vi "Control_BSA_setup.vi"(0 "setup":T1, 7 "BSA number":string) -> ()   [LabVIEW 2011]
uses:
  Controls/Setup.ctl
  Globals/LDA_meas_global_2.vi
  Globals/LDA_meas_global_1.vi
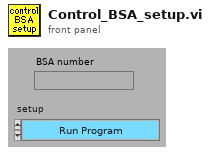
[diagram p1: front panel]
types:
  T1 = typedef "Setup.ctl" = enum16{"Run Program", "Show Setup", "Save Current Setup", "Setup Front Panel"}
  T2 = enum16{"Velocity", "Transit time", "Arrival time"}
  T3 = typedef "BSA_info_Cluster.ctl" = cluster{"GPIB Address":string, "No of Check Bytes":i32, "Extra Info":string, "COLOUR":u32, "Wavelength (nm)":dbl}
  T4 = cluster{"Output data format":enum16{"Velocity, transit time, arrival time", "Velocity, arrival time", "Velocity, transit time", "Velocity"}, "Non-validated signals":enum16{"Accept", "Reject"}}
  T5 = cluster{"High voltage":i16, "Signal gain (dB)":i16}
  T6 = enum16{"6.4", "3.2", "1.6", "0.8", "0.4", "0.2", "0.1", "0.05"}
  T7 = cluster{"Centre Velocity":u16, "Velocity span":u16, "Units":enum16{"Hz", "m/s"}, "Frequency shift":enum16{"Disabled", "Enabled"}}
  T8 = cluster{"Arrival time clock":enum16{"External", "Internal"}, "Clock source":enum16{"Slave", "Master", "Private"}, "Coincidence":enum16{"Slave", "Master", "Private"}}
  T9 = cluster{"Dead time (s)":dbl, "Duty cycle (%)":dbl, "Data collection mode":enum16{"Burst", "Contiuous", "Dead time", "External"}}
  T10 = cluster{"Burst criterion":enum16{"Envelope", "Pedestal", "Env and ped"}, "Oversize reject level":enum16{"1 (disabled)", "2", "3", "4", "5", "6", "7", "8", "9"}, "Pedestal attenuation":enum16{"0", "6", "12", "18"}, "Record length":enum16{"8", "16", "32", "64"}, "Quality factor":i16}
  T11 = cluster{"Centre frequency":u16, "Bandwidth":u16, "Units":enum16{"Hz", "m/s"}, "Frequency shift":enum16{"Disabled", "Enabled"}}
  T12 = enum16{"Velocity, transit time, arrival time", "Velocity, arrival time", "Velocity, transit time", "Velocity"}
  T13 = enum16{"Velocity", "Transit time", "Arrival time"}[]
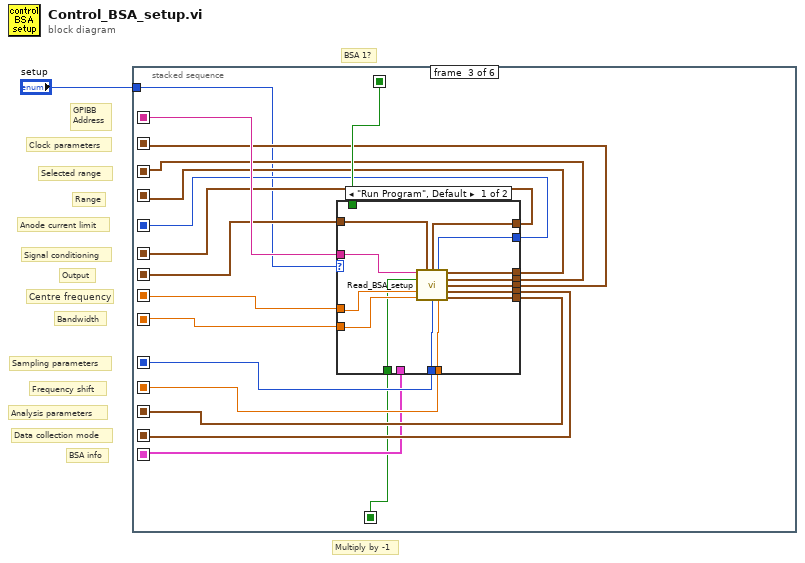
[diagram p0: block diagram]
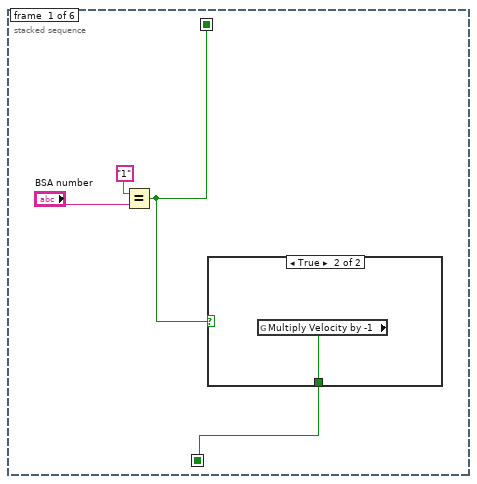
[diagram p2: hidden frame]
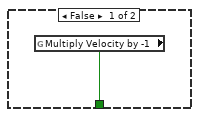
[diagram p3: hidden frame]
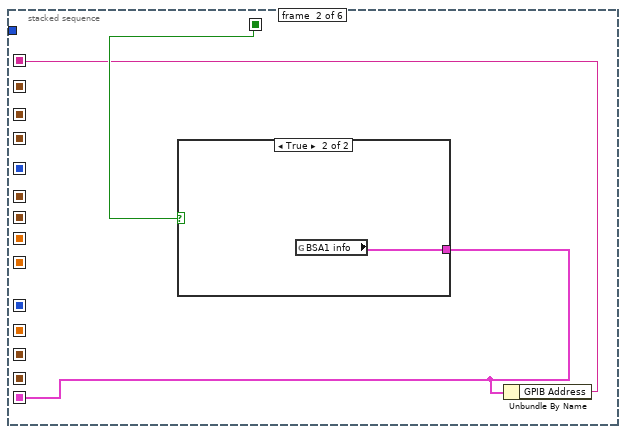
[diagram p4: hidden frame]
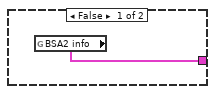
[diagram p5: hidden frame]
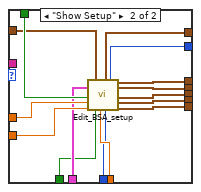
[diagram p6: hidden frame]
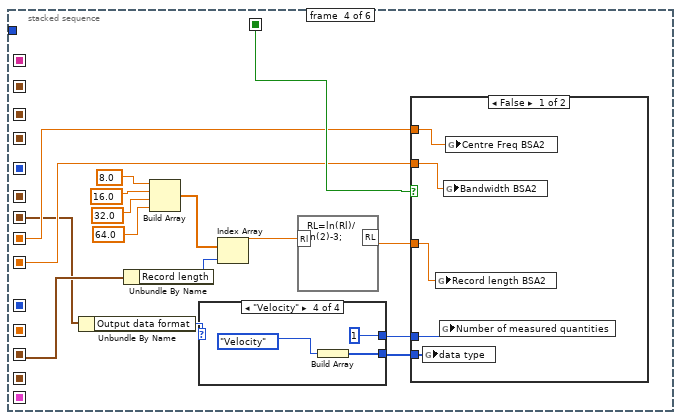
[diagram p7: hidden frame]
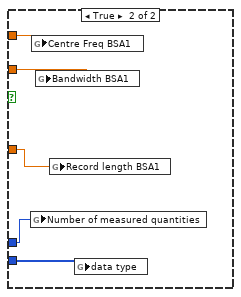
[diagram p8: hidden frame]
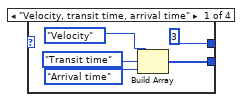
[diagram p9: hidden frame]
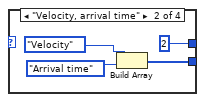
[diagram p10: hidden frame]
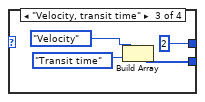
[diagram p11: hidden frame]
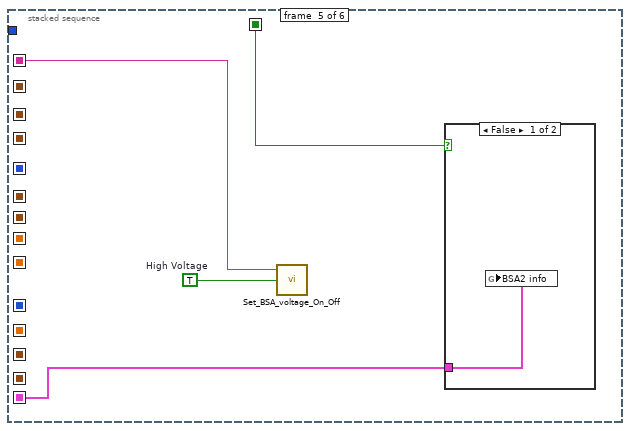
[diagram p12: hidden frame]
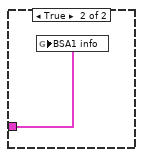
[diagram p13: hidden frame]
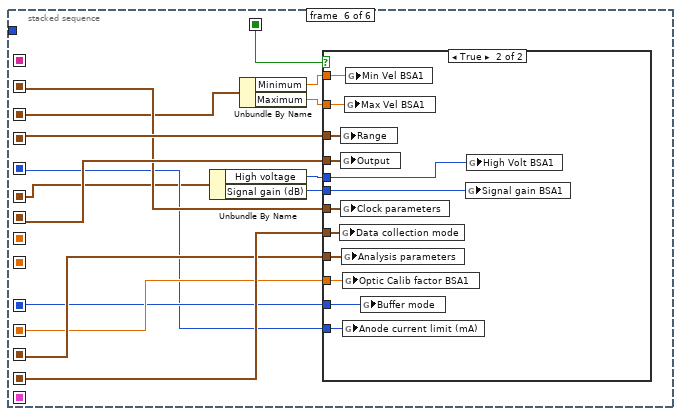
[diagram p14: hidden frame]
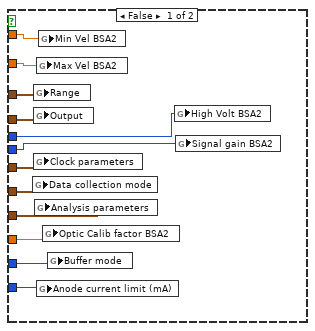
[diagram p15: hidden frame]
diagram:
  # "Multiply by -1"
  # "Bandwidth"
  # "Centre frequency"
  # "Anode current limit"
  # "Selected range"
  # "Range"
  # "Signal conditioning"
  # "Analysis parameters"
  # "Data collection mode"
  # "Frequency shift"
  # "Output"
  # "Clock parameters"
  # "Sampling parameters"
  # "BSA 1?"
  # "BSA info"
  # "GPIBB\nAddress"
  n1 = stacked-sequence {
    seq-local: [_ _ w27 _ _ _] -> [_ _ _ _ _ w117]
    seq-local: [_ w8 _ _ _ _] -> [_ _ w29 _ w101 _]
    seq-local: [_ w9 _ _ _ _] -> [_ _ w15 _ w104 _]
    seq-local: [w3 _ _ _ _ _] -> [_ w10 w28 w69 w103 w121]
    seq-local: [_ _ w20 _ _ _] -> [_ _ _ _ _ w109]
    seq-local: [_ _ w21 _ _ _] -> [_ _ _ _ _ w120]
    seq-local: [_ _ w22 _ _ _] -> [_ _ _ _ _ w113]
    seq-local: [_ _ w23 _ _ _] -> [_ _ _ _ _ w112]
    seq-local: [_ _ w24 _ _ _] -> [_ _ _ _ _ w114]
    seq-local: [_ _ w25 _ _ _] -> [_ _ _ _ _ w115]
    seq-local: [_ _ w26 _ _ _] -> [_ _ _ w66 _ w116]
    seq-local: [_ _ w19 _ _ _] -> [_ _ _ _ _ w118]
    seq-local: [_ _ w18 _ _ _] -> [_ _ _ w59 _ w119]
    seq-local: [_ _ w17 _ _ _] -> [_ _ _ w68 _ _]
    seq-local: [_ _ w16 _ _ _] -> [_ _ _ w67 _ _]
    seq-local: [w2 _ _ _ _ _] -> [_ _ w13 _ _ _]
    tunnel: "setup" -> [_ _ w14 _ _ _]
    frame #0 {
      n2 = Equal?(x="1", y="BSA number") -> (x = y?=w3:bool)
      n3 = case shown="True" w3 {
        tunnel: [w6 w7] -> w2
        frame False {
          n4 = global read "LDA_meas_global_2.vi" "Multiply Velocity by -1"() -> (w6:bool)
        }
        frame True {
          n5 = global read "LDA_meas_global_1.vi" "Multiply Velocity by -1"() -> (w7:bool)
        }
      }
    }
    frame #1 {
      n6 = case shown="True" w10 {
        tunnel: [w11 w12] -> w9
        frame False {
          n7 = global read "LDA_meas_global_2.vi" "BSA2 info"() -> (w11:T3)
        }
        frame True {
          n8 = global read "LDA_meas_global_1.vi" "BSA1 info"() -> (w12:T3)
        }
      }
      n9 = Unbundle By Name(w9) -> ("GPIB Address"=w8:string)
    }
    frame #2 {
      n10 = case shown="\"Run Program\", Default" w14 {
        tunnel: w29 -> [w43 _]
        tunnel: w28 -> [_ w58]
        tunnel: [w42 w57] -> w21
        tunnel: [w41 w56] -> w20
        tunnel: [w40 w55] -> w19
        tunnel: [w39 w54] -> w27
        tunnel: [w38 w53] -> w26
        tunnel: [w37 w52] -> w25
        tunnel: [w36 w51] -> w24
        tunnel: [w35 w50] -> w23
        tunnel: [w34 w49] -> w22
        tunnel: [w33 w48] -> w18
        tunnel: [w32 w47] -> w17
        tunnel: [w31 w46] -> w16
        tunnel: w15 -> [_ w45]
        tunnel: w13 -> [w30 w44]
        frame "Run Program", Default {
          n11 = call "Read_BSA_setup.vi"("GPIB Address"=w43, "Multiply Velocity by -1"=w30) -> ("Output"=w33:T4, "Signal conditioning"=w35:T5, "Anode current limit (mA)"=w34:T6, "Range"=w42:T7, "Selected range"=w41:cluster{"Minimum":dbl, "Maximum":dbl}, "Clock parameters"=w40:T8, "Centre frequency"=w32:dbl, "Data collection mode"=w39:T9, "Bandwidth"=w31:dbl, "Buffer mode"=w36:enum16{"One shot", "Ring", "FIFO"}, "Calibration factor"=w37:dbl, "Analysis parameters"=w38:T10)  [unwired: 1 in, 1 out]
        }
        frame "Show Setup" {
          n12 = call "Edit_BSA_setup.vi"("BSA info"=w45, "BSA 1?"=w58, "Multiply Velocity by -1"=w44) -> ("Centre frequency"=w47:dbl, "Bandwidth"=w46:dbl, "Output"=w48:T4, "Calibration factor"=w52:dbl, "Signal conditioning (out)"=w50:T5, "Buffer mode out"=w51:enum16{"One shot", "Ring", "FIFO"}, "Anode current limit (mA)"=w49:T6, "Range (out)"=w57:T11, "Selected range"=w56:cluster{"Minimum":dbl, "Maximum":dbl}, "Clock parameters (out)"=w55:T8, "Data collection mode (out)"=w54:T9, "Analysis parameters (out)"=w53:T10)  [unwired: 1 in, 4 out]
        }
      }
    }
    frame #3 {
      n13 = Unbundle By Name(w59) -> ("Output data format"=w73:T12)
      n14 = Unbundle By Name(w66) -> ("Record length"=w74:enum16{"8", "16", "32", "64"})
      n15 = Build Array(8.0, 16.0, 32.0, 64.0) -> (w61:dbl[])
      n16 = case shown="\"Velocity\"" w73 {
        tunnel: [3 2 2 1] -> w71
        tunnel: [w88 w92 w95 w99] -> w72
        frame "Velocity, transit time, arrival time" {
          n17 = Build Array(T2."Velocity", T2."Transit time", T2."Arrival time") -> (w88:T13)
        }
        frame "Velocity, arrival time" {
          n18 = Build Array(T2."Velocity", T2."Arrival time") -> (w92:T13)
        }
        frame "Velocity, transit time" {
          n19 = Build Array(T2."Velocity", T2."Transit time") -> (w95:T13)
        }
        frame "Velocity" {
          n20 = Build Array(T2."Velocity") -> (w99:T13)
        }
      }
      n21 = Index Array(array=w61, index=w74) -> (element=w60:dbl)
      n22 = formula code="RL=ln(Rl)/ln(2)-3;"("Rl"=w60) -> ("RL"=w70:dbl)
      n23 = case shown="False" w69 {
        tunnel: w68 -> [w75 w84]
        tunnel: w72 -> [w79 w83]
        tunnel: w71 -> [w78 w82]
        tunnel: w70 -> [w77 w81]
        tunnel: w67 -> [w76 w80]
        frame False {
          n24 = global write "LDA_meas_global_2.vi" "data type"(w79) -> ()
          n25 = global write "LDA_meas_global_2.vi" "Record length BSA2"(w77) -> ()
          n26 = global write "LDA_meas_global_2.vi" "Number of measured quantities"(w78) -> ()
          n27 = global write "LDA_meas_global_2.vi" "Bandwidth BSA2"(w76) -> ()
          n28 = global write "LDA_meas_global_2.vi" "Centre Freq BSA2"(w75) -> ()
        }
        frame True {
          n29 = global write "LDA_meas_global_1.vi" "Number of measured quantities"(w82) -> ()
          n30 = global write "LDA_meas_global_1.vi" "Centre Freq BSA1"(w84) -> ()
          n31 = global write "LDA_meas_global_1.vi" "Bandwidth BSA1"(w80) -> ()
          n32 = global write "LDA_meas_global_1.vi" "Record length BSA1"(w81) -> ()
          n33 = global write "LDA_meas_global_1.vi" "data type"(w83) -> ()
        }
      }
    }
    frame #4 {
      w102 = TRUE  # High Voltage
      n34 = call "Set_BSA_voltage_On_Off.vi"("GPIB address"=w101, "High Voltage"=w102) -> ()  [unwired: 1 in, 5 out]
      n35 = case shown="False" w103 {
        tunnel: w104 -> [w105 w106]
        frame False {
          n36 = global write "LDA_meas_global_2.vi" "BSA2 info"(w105) -> ()
        }
        frame True {
          n37 = global write "LDA_meas_global_1.vi" "BSA1 info"(w106) -> ()
        }
      }
    }
    frame #5 {
      n38 = Unbundle By Name(w112) -> ("High voltage"=w111:i16, "Signal gain (dB)"=w110:i16)
      n39 = Unbundle By Name(w109) -> ("Minimum"=w108:dbl, "Maximum"=w107:dbl)
      n40 = case shown="True" w121 {
        tunnel: w120 -> [w133 w145]
        tunnel: w119 -> [w132 w144]
        tunnel: w118 -> [w131 w143]
        tunnel: w117 -> [w130 w142]
        tunnel: w116 -> [w129 w141]
        tunnel: w115 -> [w128 w140]
        tunnel: w114 -> [w127 w139]
        tunnel: w113 -> [w126 w138]
        tunnel: w111 -> [w125 w137]
        tunnel: w110 -> [w124 w136]
        tunnel: w108 -> [w123 w135]
        tunnel: w107 -> [w122 w134]
        frame False {
          n41 = global write "LDA_meas_global_2.vi" "Data collection mode"(w130) -> ()
          n42 = global write "LDA_meas_global_2.vi" "Range"(w133) -> ()
          n43 = global write "LDA_meas_global_2.vi" "Output"(w132) -> ()
          n44 = global write "LDA_meas_global_2.vi" "Clock parameters"(w131) -> ()
          n45 = global write "LDA_meas_global_2.vi" "Analysis parameters"(w129) -> ()
          n46 = global write "LDA_meas_global_2.vi" "Max Vel BSA2"(w122) -> ()
          n47 = global write "LDA_meas_global_2.vi" "Anode current limit (mA)"(w126) -> ()
          n48 = global write "LDA_meas_global_2.vi" "Min Vel BSA2"(w123) -> ()
          n49 = global write "LDA_meas_global_2.vi" "Optic Calib factor BSA2"(w128) -> ()
          n50 = global write "LDA_meas_global_2.vi" "Buffer mode"(w127) -> ()
          n51 = global write "LDA_meas_global_2.vi" "High Volt BSA2"(w125) -> ()
          n52 = global write "LDA_meas_global_2.vi" "Signal gain BSA2"(w124) -> ()
        }
        frame True {
          n53 = global write "LDA_meas_global_1.vi" "Data collection mode"(w142) -> ()
          n54 = global write "LDA_meas_global_1.vi" "Range"(w145) -> ()
          n55 = global write "LDA_meas_global_1.vi" "Output"(w144) -> ()
          n56 = global write "LDA_meas_global_1.vi" "Clock parameters"(w143) -> ()
          n57 = global write "LDA_meas_global_1.vi" "Analysis parameters"(w141) -> ()
          n58 = global write "LDA_meas_global_1.vi" "Optic Calib factor BSA1"(w140) -> ()
          n59 = global write "LDA_meas_global_1.vi" "Anode current limit (mA)"(w138) -> ()
          n60 = global write "LDA_meas_global_1.vi" "Max Vel BSA1"(w134) -> ()
          n61 = global write "LDA_meas_global_1.vi" "Min Vel BSA1"(w135) -> ()
          n62 = global write "LDA_meas_global_1.vi" "Buffer mode"(w139) -> ()
          n63 = global write "LDA_meas_global_1.vi" "Signal gain BSA1"(w136) -> ()
          n64 = global write "LDA_meas_global_1.vi" "High Volt BSA1"(w137) -> ()
        }
      }
    }
  }
